vi "HAL Fix Test.vi"() -> ()   [LabVIEW 2020, in "LAF2024Q2.lvlib"]
uses:
  LAF2024Q2.lvlib
  PsuVisaSim-Fix/PsuVisaSim-Fix.lvclass
  C:/dev/lv20CE/LAF2024Q2/LAF2024Q2/PowerSupplyVisa-Fix/PowerSupplyVisa-Fix.lvclass
  Keithley230X-Fix/Keithley230X-Fix.lvclass
  PowerSupplyVisa-Fix/PowerSupplyVisa-Fix.lvclass
  C:/dev/lv20CE/LAF2024Q2/LAF2024Q2/PowerSupply-Fix/PowerSupply-Fix.lvclass
  PowerSupply-Fix/PowerSupply-Fix.lvclass
panel:
  out "error IO":errorcluster
  in  "Sim?":bool
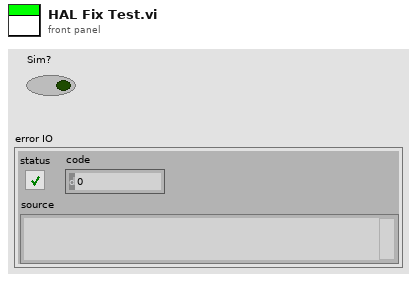
[diagram p1: front panel]
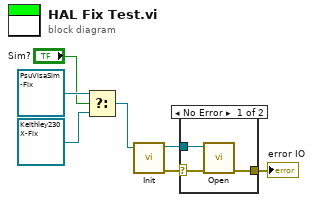
[diagram p0: block diagram]
diagram:
  n1 = Select(t=refnum<class "PsuVisaSim-Fix.lvclass"> refnum ("LAF2024Q2.lvlib:PsuVisaSim-Fix.lvclass"), s="Sim?", f=refnum<class "Keithley230X-Fix.lvclass"> refnum ("LAF2024Q2.lvlib:Keithley230X-Fix.lvclass")) -> (s? t:f=w1:refnum<class "PowerSupplyVisa-Fix.lvclass">)
  n2 = call "Init.vi"("PowerSupply-Fix in"=w1) -> ("error out"=w7:errorcluster, "PowerSupply-Fix out"=w6:refnum<class "PowerSupplyVisa-Fix.lvclass">)  [unwired: 9 in]
  n3 = case shown="No Error" w7 {
    selector: w7 -> [w9 w11]
    tunnel: w6 -> [w10 _]
    tunnel: [w8 w11] -> w5
    frame No Error {
      n4 = call "Open.vi"("error in (no error)"=w9, "PowerSupply-Fix in"=w10) -> ("error out"=w8:errorcluster)  [unwired: 8 in, 1 out]
    }
    frame Error {
    }
  }
  "error IO" <- w5
